vi "NeoPixelInit.vi"(8 "error in (no error)":errorcluster, 9 "LEDs":u8, 10 "Pin":u8, 11 "AdaFruit-Seesaw in":refnum<class "AdaFruit-Seesaw.lvclass">) -> (0 "error out":errorcluster, 3 "AdaFruit-Seesaw out":refnum<class "AdaFruit-Seesaw.lvclass">)   [LabVIEW 2020, in "CTI-Peripheral.lvlib" / "AdaFruit-Seesaw.lvclass"]
uses:
  AdaFruit-Seesaw.lvclass
  Private/SeeSawNeoPixelSpeed.ctl
  AdaFruit-Seesaw.lvclass/AdaFruit-Seesaw.ctl
  e07ed546-2582-41d2-9d86-1c81e00f0644.vi
  0e0dc425-c514-4081-9b58-af0bf55236bc.vi
  77845b78-4f67-47b5-aa9c-e7c4109e2432.vi
  0354e4dc-98d2-4c54-a780-c5ebbf35d60c.vi
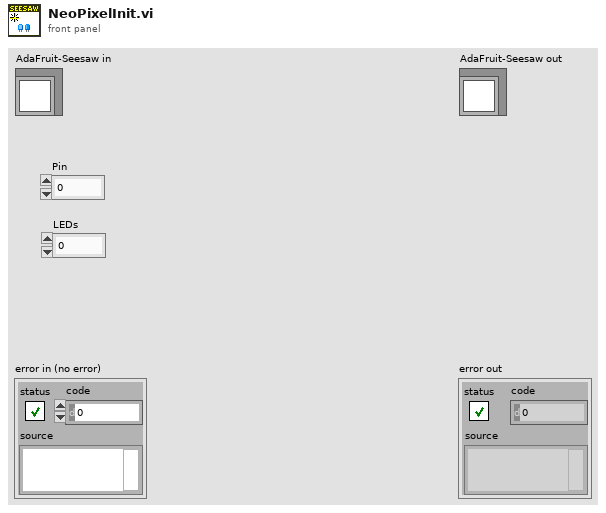
[diagram p1: front panel]
types:
  T1 = typedef "CTI-Peripheral.lvlib/AdaFruit-Seesaw.lvclass/SeeSawNeoPixelSpeed.ctl" = u8
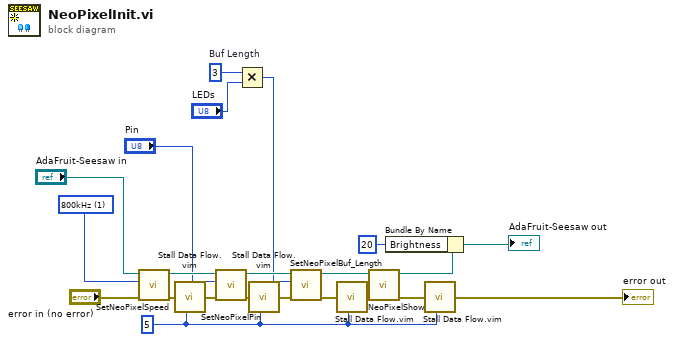
[diagram p0: block diagram]
diagram:
  w1 = u32 5 ("milliseconds to wait")
  w8 = u16 3  # Buf Length
  w17 = T1 1 items=["400kHz", "800kHz"] ("NeoPixelSpeed")
  n1 = call "SetNeoPixelSpeed.vi"("error in (no error)"="error in (no error)", "NeoPixelSpeed"=w17, "AdaFruit-Seesaw in"="AdaFruit-Seesaw in") -> ("error out"=w16:errorcluster, "AdaFruit-Seesaw out"=w21:refnum<class "AdaFruit-Seesaw.lvclass">)  [unwired: 7 in]
  n2 = call "Stall Data Flow.vim"("value in"=w16, "milliseconds to wait"=w1) -> ("value out"=w5:errorcluster)  [unwired: 1 out]
  n3 = call "SetNeoPixelPin.vi"("error in (no error)"=w5, "Pin"="Pin", "AdaFruit-Seesaw in"=w21) -> ("error out"=w15:errorcluster, "AdaFruit-Seesaw out"=w20:refnum<class "AdaFruit-Seesaw.lvclass">)  [unwired: 7 in]
  n4 = Multiply(x=w8, y="LEDs") -> (x*y=w6:u16)
  n5 = call "Stall Data Flow.vim"("value in"=w15, "milliseconds to wait"=w1) -> ("value out"=w4:errorcluster)  [unwired: 1 out]
  n6 = call "SetNeoPixelBuf_Length.vi"("error in (no error)"=w4, "Buf Length"=w6, "AdaFruit-Seesaw in"=w20) -> ("error out"=w14:errorcluster, "AdaFruit-Seesaw out"=w19:refnum<class "AdaFruit-Seesaw.lvclass">)  [unwired: 7 in]
  n7 = call "Stall Data Flow.vim"("value in"=w14, "milliseconds to wait"=w1) -> ("value out"=w3:errorcluster)  [unwired: 1 out]
  n8 = call "NeoPixelShow.vi"("error in (no error)"=w3, "AdaFruit-Seesaw in"=w19) -> ("error out"=w13:errorcluster, "AdaFruit-Seesaw out"=w11:refnum<class "AdaFruit-Seesaw.lvclass">)  [unwired: 8 in]
  n9 = Bundle By Name(cluster=w11, "Brightness"=u8 20) -> (→"AdaFruit-Seesaw out":refnum<class "AdaFruit-Seesaw.lvclass">)
  n10 = call "Stall Data Flow.vim"("value in"=w13, "milliseconds to wait"=w1) -> ("value out"=→"error out":errorcluster)  [unwired: 1 out]
